vi "test Check for Invalid Section IDs.vi"(8 "error in (no error)":errorcluster, 11 "TestCase in":refnum<class "Routing and Faulting Scripting Unit Tests.lvclass">) -> (0 "error out":errorcluster, 3 "TestCase out":refnum<class "Routing and Faulting Scripting Unit Tests.lvclass">)   [LabVIEW 2017, in "Routing and Faulting Scripting Unit Tests.lvclass"]
uses:
  Routing and Faulting Scripting Unit Tests.lvclass
  <vilib>/NI Veristand/Custom Device API/Custom Device Item Ref.ctl
  Routing and Faulting Scripting Unit Tests.lvclass/Routing and Faulting Scripting Unit Tests.ctl
  Shared/Alias Mapping.ctl
  Shared/Alias Endpoint.ctl
  <vilib>/addons/_JKI Toolkits/VI Tester/TestCase.llb/TestCase.lvclass
  Routing and Faulting Scripting.lvlib
  Shared/Routing and Faulting Shared.lvlib
  <vilib>/NI Veristand/Custom Device API/Custom Device API.lvlib
  C:/Program Files (x86)/National Instruments/LabVIEW 2017/vi.lib/addons/_JKI Toolkits/VI Tester/TestCase.llb/TestCase.lvclass
panel:
  in  "Save?":bool
  out "Output Filename":string
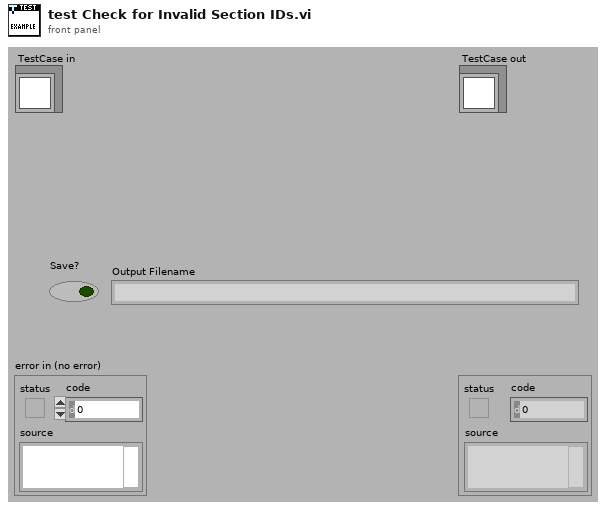
[diagram p1: front panel]
types:
  T1 = typedef "Custom Device API.lvlib/Custom Device Item Ref.ctl" = u64
  T2 = typedef "Routing and Faulting Shared.lvlib/Alias Endpoint.ctl" = cluster{"Module Path":string, "Endpoint":string}
  T3 = typedef "Routing and Faulting Shared.lvlib/Alias Mapping.ctl" = cluster{"Alias":string, "Endpoint":T2}
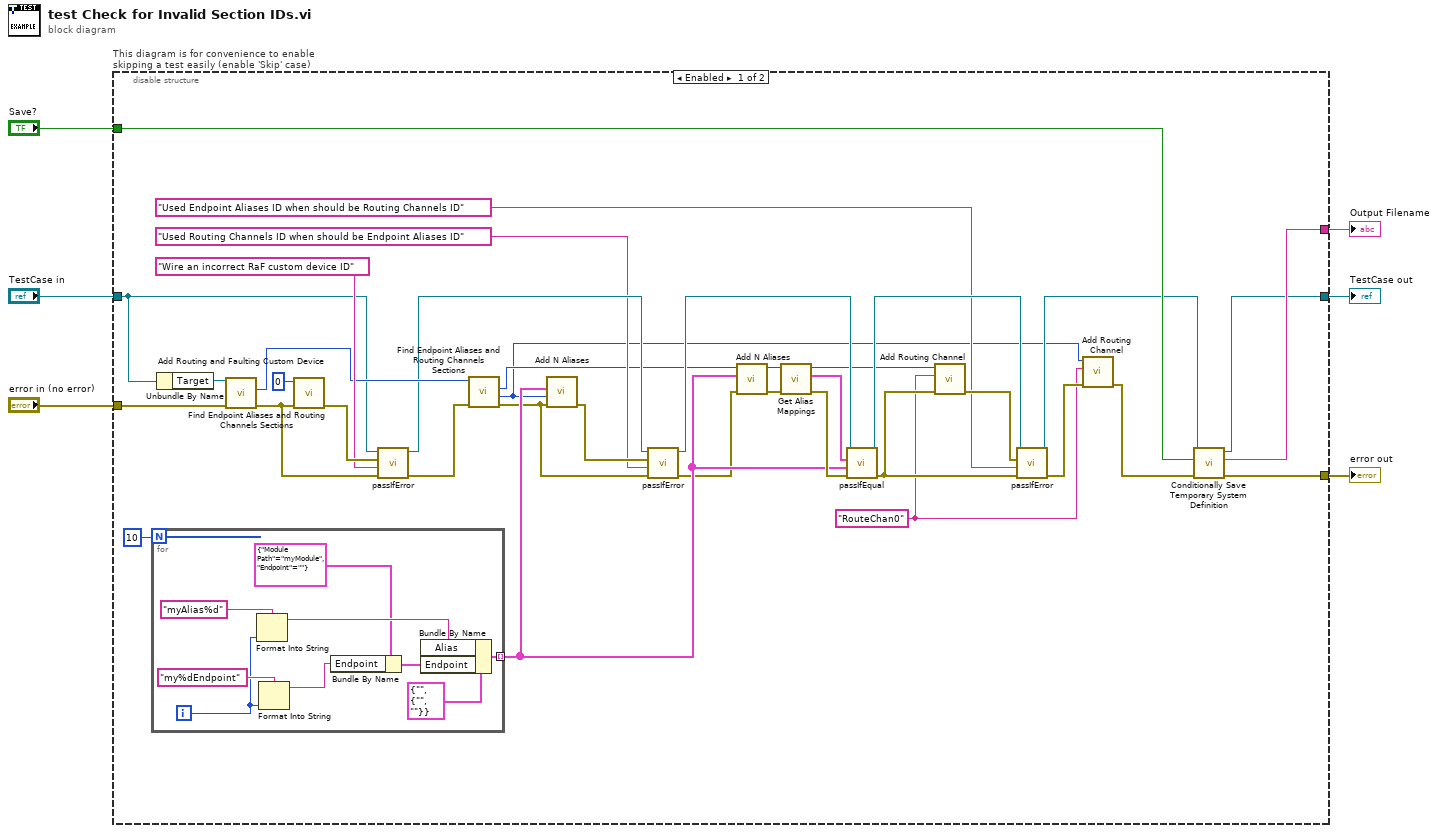
[diagram p0: block diagram]
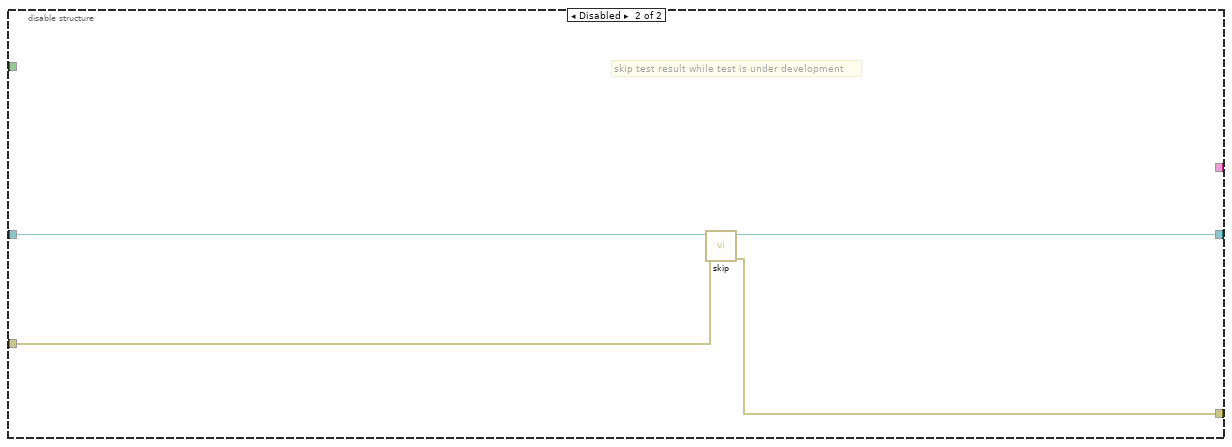
[diagram p2: hidden frame]
diagram:
  n1 = disable-structure "This diagram is for convenience to enable skipping a test easily (enable 'Skip' case)" shown="Enabled" {
    disable-tunnel: "TestCase in" -> [w25 w55]
    disable-tunnel: [w40 w53] -> w3
    disable-tunnel: [w41 w54] -> w5
    disable-tunnel: "error in (no error)" -> [w38 w52]
    disable-tunnel: [w42 _] -> w2
    disable-tunnel: "Save?" -> [w37 _]
    frame Enabled {
      w8 = "RouteChan0" ("Channel Name")
      n2 = for {
        N: 10 -> [_]
        tunnel: [w46] -> w24 mode=indexing
        i -> [w49]
        n3 = Format Into String(format string="myAlias%d" ("Alias"), w49) -> (resulting string=w47:string)  [unwired: 2 in, 1 out]
        n4 = Format Into String(format string="my%dEndpoint" ("Alias"), w49) -> (resulting string=w43:string)  [unwired: 2 in, 1 out]
        n5 = Bundle By Name(cluster=T2 {"Module Path"="myModule", "Endpoint"=""} ("Endpoint"), "Endpoint"=w43) -> (w44:T2)
        n6 = Bundle By Name(cluster=T3 {"Alias"="", "Endpoint"={"Module Path"="", "Endpoint"=""}} ("Alias Mapping"), "Alias"=w47, "Endpoint"=w44) -> (w46:T3)
      }
      n7 = Unbundle By Name(w25) -> ("Target"=w39:refnum<k24>)
      n8 = call "Add Routing and Faulting Custom Device.vi"("error in (no error)"=w38, "Target in"=w39) -> ("error out"=w31:errorcluster, "Routing and Faulting Custom Device Ref"=w28:T1)  [unwired: 7 in, 1 out]
      n9 = call "Find Endpoint Aliases and Routing Channels Sections.vi"("error in (no error)"=w31, "Routing and Faulting Custom Device Ref in"=T1 0) -> ("error out"=w30:errorcluster)  [unwired: 6 in, 3 out]
      n10 = call-dynamic "passIfError.vi"("error in (no error)"=w31, "task (\"\")"="Wire an incorrect RaF custom device ID" ("task (\"\")"), "error"=w30, "TestCase in"=w25) -> ("error out"=w27:errorcluster, "TestCase out"=w23:refnum<class "Routing and Faulting Scripting Unit Tests.lvclass">)  [unwired: 6 in]
      n11 = call "Find Endpoint Aliases and Routing Channels Sections.vi"("error in (no error)"=w27, "Routing and Faulting Custom Device Ref in"=w28) -> ("error out"=w21:errorcluster, "Routing Channels Ref"=w7:T1, "Endpoint Aliases Ref"=w17:T1)  [unwired: 6 in, 1 out]
      n12 = call "Add N Aliases.vi"("error in (no error)"=w21, "Alias Mappings"=w24, "Endpoint Aliases Ref in"=w7) -> ("error out"=w20:errorcluster)  [unwired: 7 in, 1 out]
      n13 = call-dynamic "passIfError.vi"("error in (no error)"=w21, "task (\"\")"="Used Routing Channels ID when should be Endpoint Aliases ID" ("task (\"\")"), "error"=w20, "TestCase in"=w23) -> ("error out"=w18:errorcluster, "TestCase out"=w22:refnum<class "Routing and Faulting Scripting Unit Tests.lvclass">)  [unwired: 6 in]
      n14 = call "Add N Aliases.vi"("error in (no error)"=w18, "Alias Mappings"=w24, "Endpoint Aliases Ref in"=w17) -> ("error out"=w36:errorcluster, "Endpoint Aliases Ref out"=w35:T1)  [unwired: 7 in]
      n15 = call "Get Alias Mappings.vi"("error in (no error)"=w36, "Endpoint Aliases Ref in"=w35) -> ("error out"=w34:errorcluster, "Alias Mappings"=w33:T3[], "Endpoint Aliases Ref out"=w12:T1)  [unwired: 7 in]
      n16 = call-dynamic "passIfEqual.vi"("error in (no error)"=w34, "y"=w24, "x"=w33, "TestCase in"=w22) -> ("error out"=w14:errorcluster, "TestCase out"=w16:refnum<class "Routing and Faulting Scripting Unit Tests.lvclass">)  [unwired: 6 in]
      n17 = call "Add Routing Channel.vi"("error in (no error)"=w14, "Channel Name"=w8, "Routing Channels Ref in"=w12) -> ("error out"=w13:errorcluster)  [unwired: 6 in, 2 out]
      n18 = call-dynamic "passIfError.vi"("error in (no error)"=w14, "task (\"\")"="Used Endpoint Aliases ID when should be Routing Channels ID" ("task (\"\")"), "error"=w13, "TestCase in"=w16) -> ("error out"=w10:errorcluster, "TestCase out"=w15:refnum<class "Routing and Faulting Scripting Unit Tests.lvclass">)  [unwired: 6 in]
      n19 = call "Add Routing Channel.vi"("error in (no error)"=w10, "Channel Name"=w8, "Routing Channels Ref in"=w7) -> ("error out"=w9:errorcluster)  [unwired: 6 in, 2 out]
      n20 = call "Conditionally Save Temporary System Definition.vi"("error in (no error)"=w9, "Save?"=w37, "Test Case"=w15) -> ("error out"=w41:errorcluster, "filename"=w42:string, "Test Case"=w40:refnum<class "Routing and Faulting Scripting Unit Tests.lvclass">)  [unwired: 6 in]
    }
    frame Disabled {
      # "skip test result while test is under development"
      n21 = call <vilib>:"skip.vi"("error in (no error)"=w52, "TestCase in"=w55) -> ("error out"=w54:errorcluster, "TestCase out"=w53:refnum<class "Routing and Faulting Scripting Unit Tests.lvclass">)  [unwired: 8 in]
    }
  }
  "error out" <- w5
  "TestCase out" <- w3
  "Output Filename" <- w2
